vi "Tegam4040 - Gain.vi"(0 "Instrument Session Handle In":u32 format="%x", 1 "Gain":enum16{"Gain of 1", "Gain of 10", "Gain of 100"}(ring), 11 "error in (no error)":errorcluster) -> (4 "Instrument Session Handle Out (dupl)":u32 format="%x", 15 "error out":errorcluster)   [LabVIEW 2010, in "Tegam4040.lvlib"]
doc: "Gain Stage: Bits 6-8.\n\n0: Gain set to 1\n1: Gain set to 10\n2: Gain set to 100\n\n\nCalibration bit will be reset if attuation is changed."
uses:
  Tegam4040.lvlib
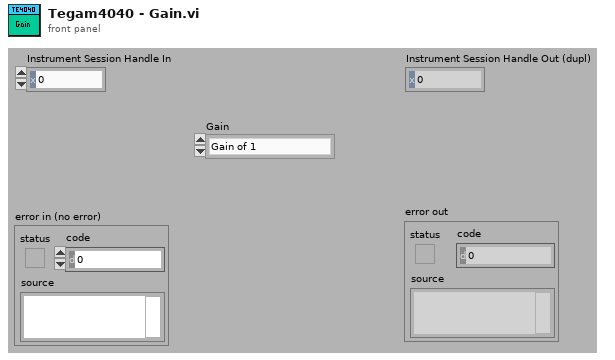
[diagram p1: front panel]
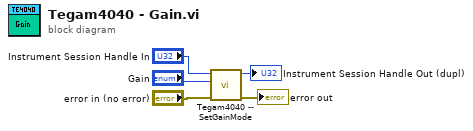
[diagram p0: block diagram]
diagram:
  n1 = call "Tegam4040 -- SetGainMode.vi"("error in (no error)"="error in (no error)", "Gain"="Gain", "Instrument Session Handle In"="Instrument Session Handle In") -> ("error out"=→"error out":errorcluster, "Instrument Session Handle Out (dupl)"=→"Instrument Session Handle Out (dupl)":u32)  [unwired: 7 in]
